vi "Test Method Status Reset on Start.vi"(8 "error in (no error)":errorcluster, 11 "Result Model Result Recording Test in":refnum<class "Result Model Result Recording Test.lvclass">) -> (0 "error out":errorcluster, 3 "Result Model Result Recording Test out":refnum<class "Result Model Result Recording Test.lvclass">)   [LabVIEW 2020, in "Result Model Result Recording Test.lvclass"]
uses:
  Result Model Result Recording Test.lvclass
  source/Core/Result/Type.ctl
  source/Core/Result/Result.lvlib
  source/Core/Result/Status.ctl
  source/Core/Result/Result.ctl
  ae2c71b8-32bb-49d1-8500-0119bfec74ff.vi
  source/User Interface/Result Model/Result Model.lvclass
  source/User Interface/Result Model/Tree Item Filter.ctl
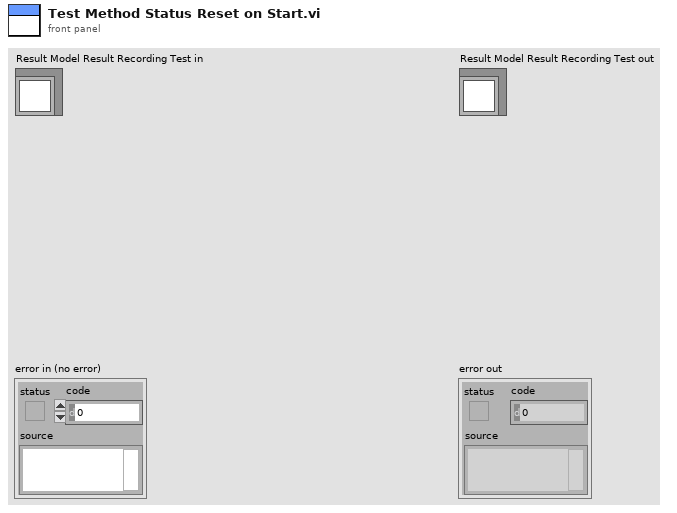
[diagram p1: front panel]
types:
  T1 = typedef "Result Model.lvclass/Tree Item Filter.ctl" = enum16{"All", "Only Fails", "Fails or else Not Executed"}
  T2 = typedef "Result.lvlib/Result.ctl" = cluster{"Name":string, "Description":string, "Status":T3, "Result Type":T4, "Execution Time":dbl, "Data":cluster{"Expected":variant, "Actual":variant, "Delta":variant}}
  T3 = typedef "Result.lvlib/Status.ctl" = enum16{"", "Passed", "Failed", "Error", "Skipped", "Setup Error", "Broken", "Teardown Error"}
  T4 = typedef "Result.lvlib/Type.ctl" = enum16{"Test Case", "Test Suite", "Test Run", "Pass", "Fail", "Skip", "Pass if", "Fail if", "Pass if Error", "Fail if Error", "Pass if Equal", "Fail if Equal"}
  T5 = cluster{"Left Cell String":string, "Child Text":string[], "Child Tag":string, "Item Indent":i32, "Child Only?":bool, "Glyph Index":i32}[]
  T6 = cluster{"Left Cell String":string, "Child Text":string[], "Child Tag":string, "Item Indent":i32, "Child Only?":bool, "Glyph Index":i32}
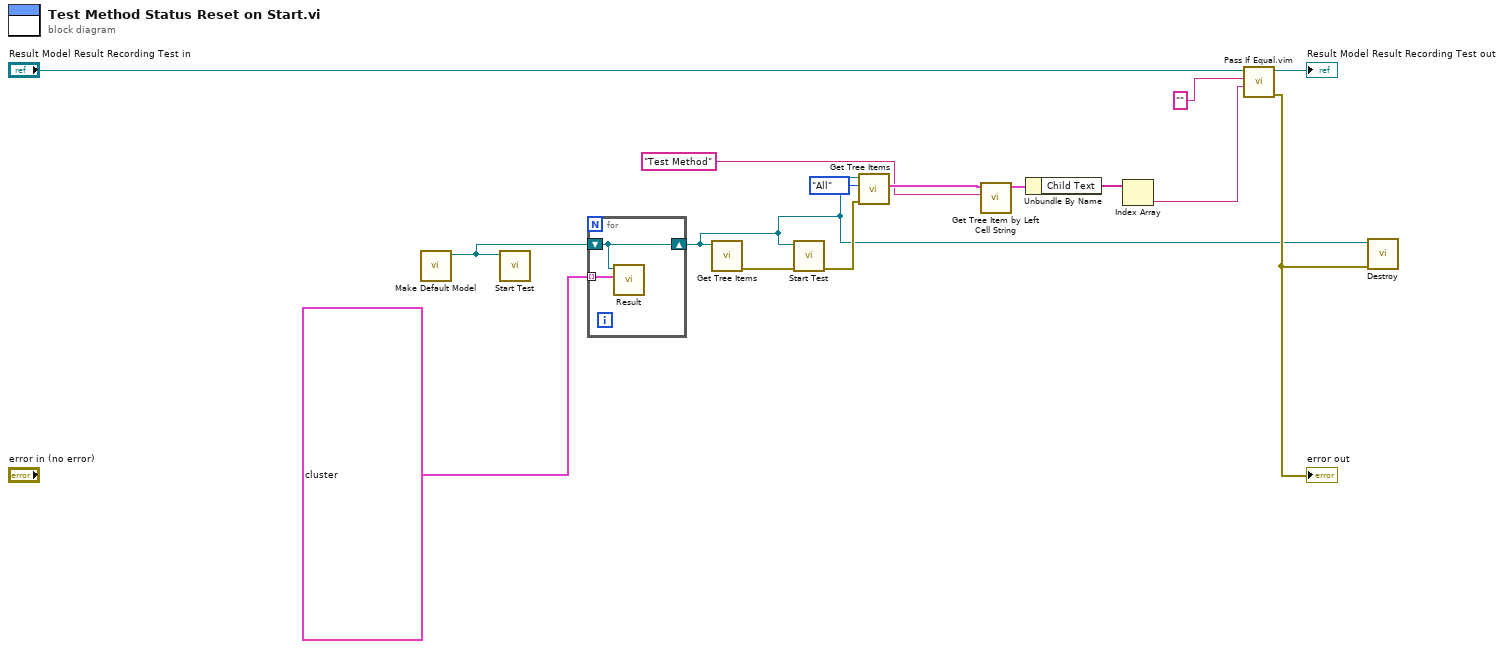
[diagram p0: block diagram]
diagram:
  n1 = call "Make Default Model.vi"() -> ("Result Model out"=w4:refnum<class "Result Model.lvclass">)  [unwired: 10 in, 1 out]
  n2 = call "Start Test.vi"("Result Model by Reference In"=w4) -> ()  [unwired: 10 in, 1 out]
  n3 = for {
    tunnel: T2[] [{"Name"="Case.lvclass:Test Method.vi", "Description"="Failed:\nMessage", "Status"=enum."Failed", "Result Type"=enum."Pass", "Execution Time"=0.107, "Data"={"Expected"=variant, "Actual"=variant, "Delta"=variant}}, {"Name"="Case.lvclass:Test Method.vi", "Description"="", "Status"=enum."Passed", "Result Type"=enum."Test Case", "Execution Time"=0.0, "Data"={"Expected"=variant, "Actual"=variant, "Delta"=variant}}] ("Results") -> [w17] mode=indexing
    shift-right: [w16] -> w2
    shift-left: w4 -> [w16]
    n4 = call-dynamic "Result.vi"("Results"=w17, "Result Model by Reference In"=w16) -> ()  [unwired: 9 in, 1 out]
  }
  n5 = call "Get Tree Items.vi"("Result Model by Reference In"=w2) -> ("error out"=w1:errorcluster)  [unwired: 9 in, 1 out]
  n6 = call "Start Test.vi"("error in (no error)"=w1, "Result Model by Reference In"=w2) -> ("error out"=w3:errorcluster)  [unwired: 9 in]
  n7 = call "Get Tree Items.vi"("error in (no error)"=w3, "Filter"=Tree_Item_Filter."All", "Result Model by Reference In"=w2) -> ("Tree Items"=w12:T5)  [unwired: 7 in, 1 out]
  n8 = call "Get Tree Item by Left Cell String.vi"("Left Cell String"="Test Method" ("Item"), "Tree Items"=w12) -> ("Item"=w10:T6)  [unwired: 9 in]
  n9 = Unbundle By Name(w10) -> ("Child Text"=w9:string[])
  n10 = Index Array(array=w9) -> (element=w8:string)  [unwired: 1 in]
  n11 = call "Pass If Equal.vim"("Actual"=w8, "Expected"="" ("element"), "LUnit Test Case In"="Result Model Result Recording Test in") -> ("error out"=w5:errorcluster, "LUnit Test Case Out"=→"Result Model Result Recording Test out":refnum<class "Result Model Result Recording Test.lvclass">)  [unwired: 7 in]
  "error out" <- w5
  n12 = call "Destroy.vi"("error in (no error)"=w5, "Result Model in"=w2) -> ()  [unwired: 9 in, 1 out]
